vi "NumberOfPhases.vi"(11 "Device(s) Settings":T1 {"Waveform"."Waveform (1: Sine)" items=["Sine"=1, "Arbitrary Waveform 2"=2, "Arbitrary Waveform 3"=3, "Arbitrary Waveform 4"=4, "Arbitrary Waveform 5"=5, "Arbitrary Waveform 6"=6, "Arbitrary Waveform 7"=7, "Arbitrary Waveform 8"=8, "Arbitrary Waveform 9"=9, "Arbitrary Waveform 10"=10, "Arbitrary Waveform 11"=11, "Arbitrary Waveform 12"=12, "Arbitrary Waveform 13"=13, "Arbitrary Waveform 14"=14, "Arbitrary Waveform 15"=15, "Arbitrary Waveform 16"=16, "Arbitrary Waveform 17"=17, "Arbitrary Waveform 18"=18, "Arbitrary Waveform 19"=19, "Arbitrary Waveform 20"=20, "Arbitrary Waveform 21"=21, "Arbitrary Waveform 22"=22]; "Waveform"."Channel Name (1: A)" items=["A"=1, "B"=2, "C"=3]; "Configure Output"."Form (3: Three)" items=["Single"=1, "Split"=2, "Three"=3]; "Configure Output"."Coupling  (0: Direct)" items=["Direct", "Transformer"]; "Source Limits and Range"."Frequency Range (600Hz)" items=["150 Hz", "300 Hz", "600 Hz", "1200 Hz"]; "Source Limits and Range"."Range Control (0: Auto)" items=["Auto", "<110 V", "110 V -120.9 V", "121 V - 130.9 V", "> 131 V"]}) -> (2 "Numeric Indicator":i32, 3 "Error Out":errorcluster, 5 "Boolean":bool)   [LabVIEW 2018, in "AcPwrPlugins.lvlib" / "PacificPowerSource.lvclass"]
uses:
  PacificPowerSource.lvclass
  TypeDefs/DeviceSettings.ctl
  <vilib>/Utility/error.llb/Error Cluster From Error Code.vi
  <vilib>/ErrorRing/Error Ring.xnode
panel:
  in  "Error In":errorcluster
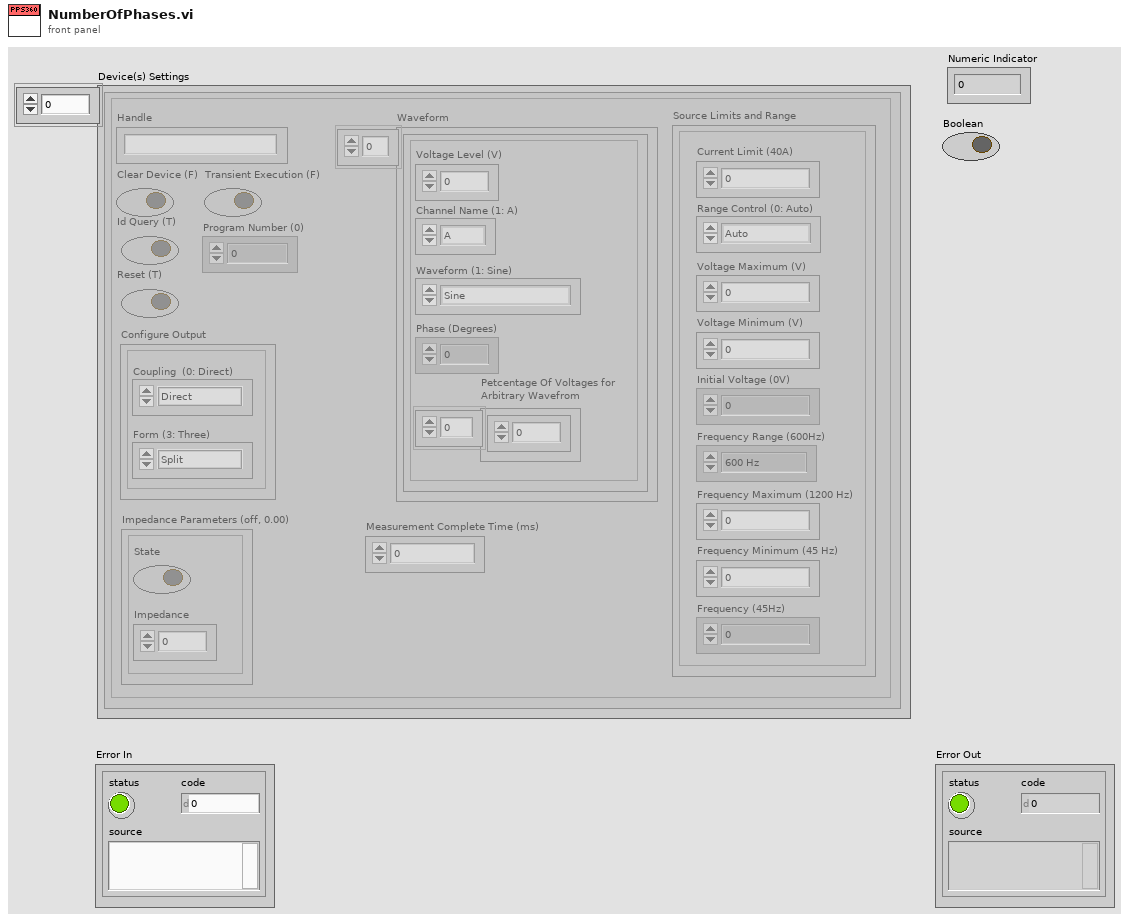
[diagram p1: front panel]
types:
  T1 = typedef "AcPwrPlugins.lvlib/PacificPowerSource.lvclass/DeviceSettings.ctl" = cluster{"Handle":string, "Connected":bool, "Source Limits and Range":cluster{"Frequency Minimum (45 Hz)":dbl, "Frequency Maximum (1200 Hz)":dbl, "Voltage Maximum (V)":dbl, "Voltage Minimum (V)":dbl, "Current Limit (40A)":dbl, "Range Control (0: Auto)":u16, "Initial Voltage (0V)":u16, "Frequency Range (600Hz)":u16, "Frequency (45Hz)":dbl}, "Clear Device (F)":bool, "Configure Output":cluster{"Coupling  (0: Direct)":u16, "Form (3: Three)":u16}, "btnIdQuery":bool, "btnReset":bool, "Waveform":cluster{"Voltage Level (V)":dbl, "Phase (Degrees)":i32, "Channel Name (1: A)":u16, "Waveform (1: Sine)":u16, "Petcentage Of Voltages for \nArbitrary Wavefrom":dbl[]}[], "Impedance Parameters (off, 0.00)":cluster{"State":bool, "Impedance":dbl}, "Program Number (0)":i32, "Transient Execution (F)":bool, "OutputEnabled":bool, "Measurement Complete Time (ms)":u32}[]
  T2 = cluster{"Voltage Level (V)":dbl, "Phase (Degrees)":i32, "Channel Name (1: A)":u16, "Waveform (1: Sine)":u16, "Petcentage Of Voltages for \nArbitrary Wavefrom":dbl[]}[]
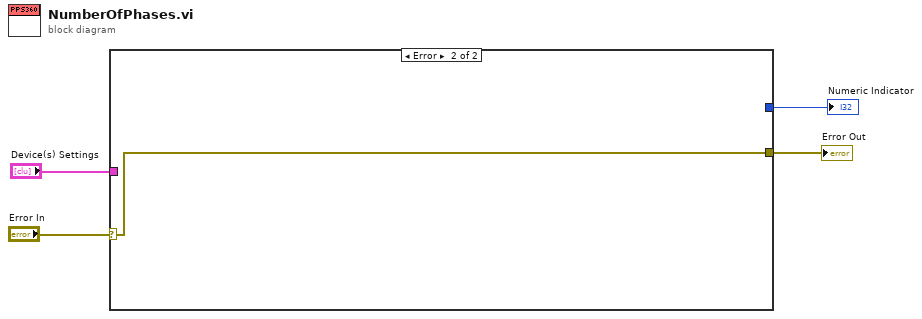
[diagram p0: block diagram]
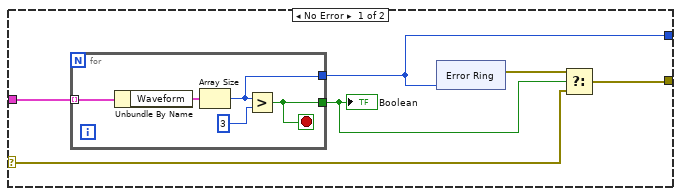
[diagram p2: hidden frame]
diagram:
  n1 = case shown="Error" "Error In" {
    selector: "Error In" -> [w5 w23]
    tunnel: "Device(s) Settings" -> [w10 _]
    tunnel: [w9 _] -> w3
    tunnel: [w7 w23] -> w2
    frame No Error {
      n2 = for {
        tunnel: w10 -> [w20] mode=indexing
        tunnel: [w19] -> w6
        tunnel: [w18] -> w9
        stop <- w19 stop-if-true
        n3 = Unbundle By Name(w20) -> ("Waveform"=w22:T2)
        n4 = Array Size(array=w22) -> (size(s)=w18:i32)
        n5 = Greater?(x=w18, y=3) -> (0:w19:bool)
      }
      "Boolean" <- w6
      n6 = xnode "Error Ring"("parameter 0"=w9) -> ("error out"=w8:errorcluster)
      n7 = Select(t=w8, s=w6, f=w5) -> (s? t:f=w7:errorcluster)
    }
    frame Error {
    }
  }
  "Numeric Indicator" <- w3
  "Error Out" <- w2
